vi "AD7609 sleepmode.vi"(1 "Sleep state":u8(ring) items=["Awake", "Standby", "Shutdown"]) -> (0 "Sleep error out":errorcluster)   [LabVIEW 2015]
uses:
  <vilib>/Instr/_visa.llb/VISA Open Access Mode.ctl
  AD7609 global.vi
panel:
  out "Sleep string output":string
  # "PN 25/11/2014, 17/08/2015"
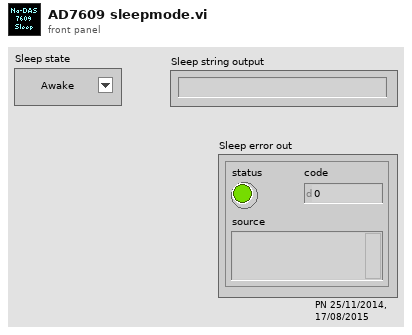
[diagram p1: front panel]
types:
  T1 = typedef "VISA Open Access Mode.ctl" = u32
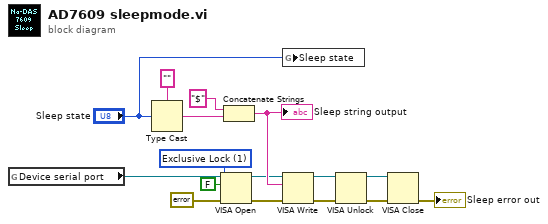
[diagram p0: block diagram]
diagram:
  w12 = T1 1 items=["VISA Defaults"=0, "Exclusive Lock"=1, "Load Configured Settings"=4] ("Access Mode")
  n1 = global read "AD7609 global.vi" "Device serial port"() -> (w4:refnum<visa-resource-name>)
  n2 = Type Cast(type="", x="Sleep state") -> (*(type *) &x=w15:string)
  n3 = VISA Open(duplicate session (F)=FALSE, access mode=w12, error in (no error)=errorcluster {"status"=FALSE, "code"=0, "source"=""}, VISA resource name=w4) -> (VISA resource name=w2:refnum<visa-resource-name>, error out=w1:errorcluster)  [unwired: 1 in]
  n4 = Concatenate Strings("$", w15) -> (w13:string)
  "Sleep string output" <- w13
  n5 = global write "AD7609 global.vi" "Sleep state"("Sleep state") -> ()
  n6 = VISA Write(VISA resource name=w2, write buffer=w13, error in (no error)=w1) -> (VISA resource name out=w7:refnum<visa-resource-name>, error out=w6:errorcluster)  [unwired: 1 out]
  n7 = VISA Unlock(8:w6, 11:w7) -> (0:w9:errorcluster, 3:w10:refnum<visa-resource-name>)
  n8 = VISA Close(VISA resource name=w10, error in (no error)=w9) -> (error out=→"Sleep error out":errorcluster)
